vi "Load.vi"(8 "error in (no error)":errorcluster, 10 "Path":path, 11 "XML in":refnum<class "XML.lvclass">) -> (0 "error out":errorcluster, 3 "XML out":refnum<class "XML.lvclass">, 5 "Flattened String":string)   [LabVIEW 2020, in "XML.lvlib" / "XML.lvclass"]
uses:
  <vilib>/gpm_packages/@cs/persistence/source/XML/XML.lvclass
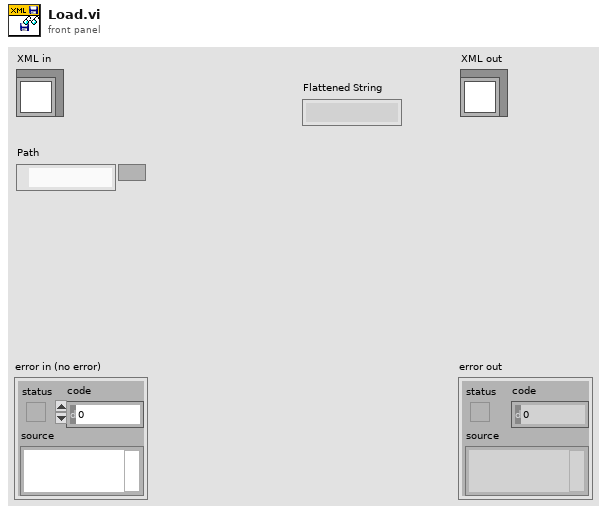
[diagram p1: front panel]
types:
  T1 = enum16{"open", "replace", "create", "open or create", "replace or create", "replace or create with confirmation"}
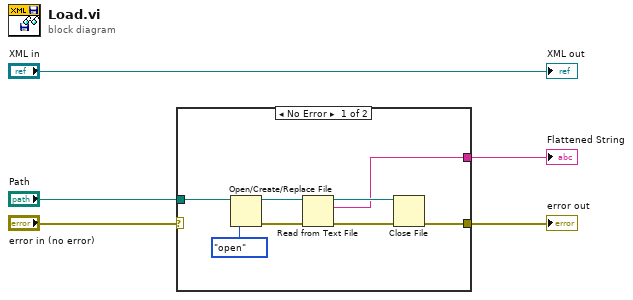
[diagram p0: block diagram]
diagram:
  n1 = case shown="No Error" "error in (no error)" {
    selector: "error in (no error)" -> [_ w14]
    tunnel: [w8 w14] -> w3
    tunnel: "Path" -> [w7 _]
    tunnel: [w6 _] -> w1
    frame No Error {
      n2 = Open/Create/Replace File(file path (use dialog)=w7, operation (0:open)=T1."open") -> (refnum out=w10:refnum<file>, error out=w12:errorcluster)  [unwired: 4 in, 1 out]
      n3 = Read from Text File(file (use dialog)=w10, error in=w12) -> (refnum out=w11:refnum<file>, text=w6:string, error out=w13:errorcluster)  [unwired: 2 in, 1 out]
      n4 = Close File(refnum=w11, error in=w13) -> (error out=w8:errorcluster)  [unwired: 1 out]
    }
    frame Error {
    }
  }
  "error out" <- w3
  "Flattened String" <- w1
  "XML out" <- "XML in"
